vi "HeaderAction.vi"(0 "DefaultDevIn":refnum<class "LeafMagnetometer.lvclass"> caption="DNL_LabVIEW Object in", 11 "error in (no error)":errorcluster caption="entrée d'erreur (pas d'erreur)") -> (4 "DefaultDevOut":refnum<class "LeafMagnetometer.lvclass"> caption="DNL_LabVIEW Object out", 6 "DataNames":string[](array[string]), 8 "Instr Name":string, 10 "HeaderString":string, 13 "ArrDisplayNames":string[](array[string]), 14 "DisplayNames":string[](array[string]), 15 "error out":errorcluster caption="sortie d'erreur")   [LabVIEW 2019, in "LeafMagnetometer.lvclass"]
uses:
  LeafMagnetometer.lvclass
  C:/Programmes Labview/LabScanV1A/DevicesClass/BaseDevice/BaseDevice.lvclass
  LeafMagnetometer.lvclass/LeafMagnetometer.ctl
  BaseDevice/BaseDevice.lvclass
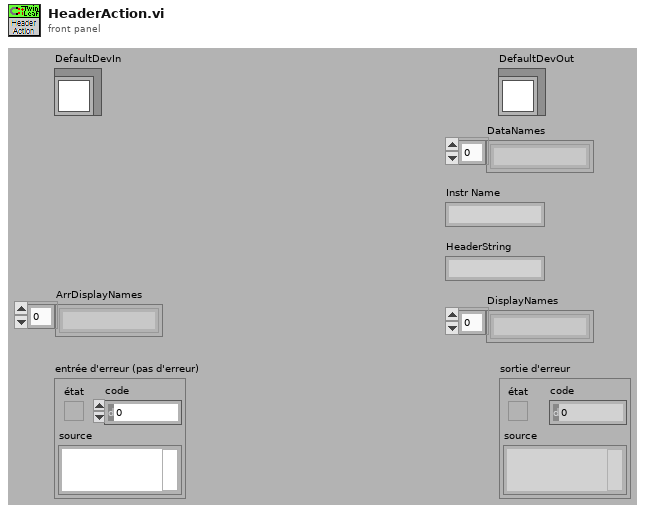
[diagram p1: front panel]
types:
  T1 = typedef "LeafMagnetometer.lvclass/LeafMagnetometer_Func.ctl" = enum16{"Read Fields (nT,nT,nT,nT)", "Read AVM Fields (nT)"}
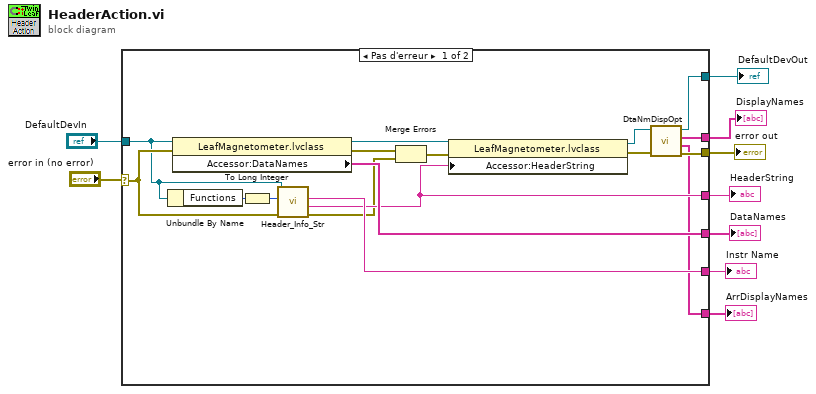
[diagram p0: block diagram]
diagram:
  n1 = case shown="Pas d'erreur" "error in (no error)" {
    selector: "error in (no error)" -> [w18 w27]
    tunnel: [w14 _] -> w8
    tunnel: [w26 _] -> w7
    tunnel: "DefaultDevIn" -> [w17 w28]
    tunnel: [w23 w27] -> w5
    tunnel: [w20 w28] -> w4
    tunnel: [w15 _] -> w3
    tunnel: [w19 _] -> w2
    tunnel: [w10 _] -> w1
    frame No Error {
      n2 = Unbundle By Name(w17) -> ("Functions"=w16:T1)
      n3 = property class="LeafMagnetometer.lvclass"(reference=w17, error in=w18) -> (reference out=w25:refnum<class "LeafMagnetometer.lvclass">, error out=w24:errorcluster, "Accessor:DataNames"=w26:string[])
      n4 = To Long Integer(number=w16) -> (32bit integer=w11:i32)
      n5 = call-dynamic "Header_Info_Str.vi"("error in (no error)"=w18, "Functions"=w11, "DefaultDev in"=w17) -> ("error out"=w12:errorcluster, "HdrInfoStr"=w14:string, "InstrumentName"=w15:string)  [unwired: 5 in, 1 out]
      n6 = Merge Errors(w24, w12) -> (w13:errorcluster)
      n7 = property class="LeafMagnetometer.lvclass"(reference=w25, error in=w13, "Accessor:HeaderString"=w14) -> (reference out=w21:refnum<class "LeafMagnetometer.lvclass">, error out=w22:errorcluster)
      n8 = call "DtaNmDispOpt.vi"("error in (no error)"=w22, "BaseDevice en entrée"=w21) -> ("error out"=w23:errorcluster, "ArrDisplayNames"=w10:string[], "DisplayNames"=w19:string[], "BaseDevice en sortie"=w20:refnum<class "LeafMagnetometer.lvclass">)  [unwired: 6 in]
    }
    frame Error {
    }
  }
  "error out" <- w5
  "DefaultDevOut" <- w4
  "DataNames" <- w7
  "HeaderString" <- w8
  "Instr Name" <- w3
  "DisplayNames" <- w2
  "ArrDisplayNames" <- w1
